vi "S2C_FORNAX_Poly_DftAudioPlayCommand.vi"(8 "Error In":errorcluster, 10 "DftAudioPlayCommand":T4={"Partition"="Default", "Message"="DftAudioPlayCommand", "M_AudioSequence"=0, "M_PlayMode"=0, "M_Priority"=0, "M_OverrideSeqVolume"=FALSE, "M_Volume"=0} {"M_Priority" items=["AUDIO_REPLACE", "AUDIO_DELAY", "AUDIO_INTRPT", "AUDIO_NO_ACT", "AUDIO_ALARM", "AUDIO_DEFAULT"]; "M_PlayMode" items=["AUDIO_MODE_CONTINUOUS", "AUDIO_MODE_ONE_TIME", "AUDIO_MODE_STOP", "AUDIO_MODE_DEFAULT"]; "M_AudioSequence" items=["AUDIO_SEQUENCE_NOT_USED", "AUDIO_SEQUENCE_SELF_TEST", "AUDIO_SEQUENCE_INSTRUMENT_INSTALLED", "AUDIO_SEQUENCE_CHANGEABLE_OPTION", "AUDIO_SEQUENCE_NON_CHANGEABLE_OPTION", "AUDIO_SEQUENCE_INVALID_SELECTION", "AUDIO_SEQUENCE_CUT_ACTIVATION", "AUDIO_SEQUENCE_DWH_ACTIVATION", "AUDIO_SEQUENCE_COAG_BIPOLAR_ACTIVATION", "AUDIO_SEQUENCE_LIGASURE_ACTIVATION", "AUDIO_SEQUENCE_INVALID_ACTIVATION", "AUDIO_SEQUENCE_SLIDER_BARS_1_TO_2", "AUDIO_SEQUENCE_SLIDER_BARS_2_TO_3", "AUDIO_SEQUENCE_SLIDER_BARS_3_TO_4", "AUDIO_SEQUENCE_SLIDER_BARS_4_TO_5", "AUDIO_SEQUENCE_SLIDER_BARS_5_TO_4", "AUDIO_SEQUENCE_SLIDER_BARS_4_TO_3", "AUDIO_SEQUENCE_SLIDER_BARS_3_TO_2", "AUDIO_SEQUENCE_SLIDER_BARS_2_TO_1", "AUDIO_SEQUENCE_VIRTUAL_AMMETER", "AUDIO_SEQUENCE_SEAL_COMPLETE", "AUDIO_SEQUENCE_INCOMPLETE_SEAL_CYCLE", "AUDIO_SEQUENCE_HIGH_ALARM", "AUDIO_SEQUENCE_MEDIUM_ALARM", "AUDIO_SEQUENCE_LOW_ALARM", "AUDIO_SEQUENCE_REM", "AUDIO_SEQUENCE_SHARED_COAG", "AUDIO_SEQUENCE_INFO", "AUDIO_SEQUENCE_CARDIOBLATE_MONO", "AUDIO_SEQUENCE_CARDIOBLATE_BIPOLAR", "AUDIO_SEQUENCE_CARDIOBLATE_TRANSMURAL", "AUDIO_SEQUENCE_CARDIOBLATE_IMPEDANCE_EXCEEDED", "AUDIO_SEQUENCE_VALLEY_ENDO", "NUM_AUDIO_SEQUENCES"]}, 11 "Settings":T5={"Driver"="Fornax", "Command"="DftAudioPlayCommand", "Return"="ErrorStatus", "Parameters"="", "Timeout"=10.0}) -> (0 "Error Out":errorcluster, 3 "Response":string)   [LabVIEW 2015]
uses:
  Typedefs/AudioSequence.ctl
  Typedefs/AudioMode.ctl
  Typedefs/AudioPriority.ctl
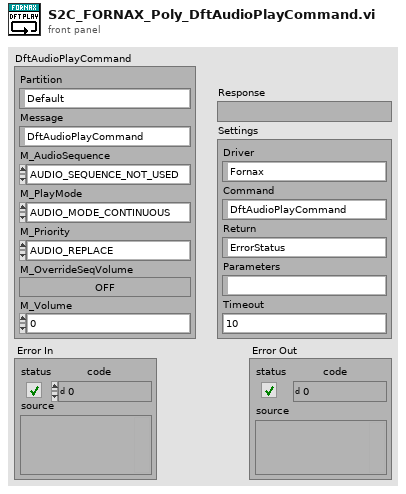
[diagram p1: front panel]
types:
  T1 = typedef "AudioSequence.ctl" = i16
  T2 = typedef "AudioMode.ctl" = i16
  T3 = typedef "AudioPriority.ctl" = i16
  T4 = cluster{"Partition":string, "Message":string, "M_AudioSequence":T1, "M_PlayMode":T2, "M_Priority":T3, "M_OverrideSeqVolume":bool, "M_Volume":i32}
  T5 = cluster{"Driver":string, "Command":string, "Return":string, "Parameters":string, "Timeout":dbl}
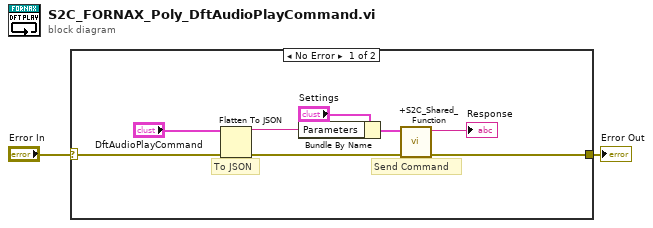
[diagram p0: block diagram]
diagram:
  n1 = case shown="No Error" "Error In" {
    selector: "Error In" -> [w6 w11]
    tunnel: [w5 w11] -> w1
    frame No Error {
      # "To JSON"
      # "Send Command"
      n2 = Flatten To JSON(anything="DftAudioPlayCommand", error in (no error)=w6) -> (JSON string=w7:string, 11:w9:errorcluster)  [unwired: 1 in]
      n3 = Bundle By Name(cluster="Settings", "Parameters"=w7) -> (w10:T5)
      n4 = call "+S2C_Shared_Function.vi"("Error In"=w9, "Settings"=w10) -> ("Error Out"=w5:errorcluster, "Response"=→"Response":string)  [unwired: 8 in]
    }
    frame Error {
    }
  }
  "Error Out" <- w1
